vi "RT Loop - System Health and Monitoring.vi"(11 "Message Queue":refnum<queue> caption="消息队列") -> ()   [LabVIEW 2013]
uses:
  support/Message Queue/Message Cluster.ctl
  Globals/Global - Configuration Options.vi
  <vilib>/nisyscfg/Close (System).vi
  Globals/Global - All RT Loop Stop.vi
  Globals/Global - Monitoring Variables.vi
  <vilib>/NI_Real-Time Target Support.lvlib
  <vilib>/nisyscfg/nisyscfg.lvlib
  <resource>/objmgr/nisysapi.rc
  support/Message Queue/Message Queue.lvlib
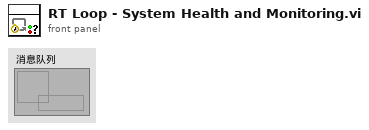
[diagram p1: front panel]
types:
  T1 = typedef "NI_Real-Time Target Support.lvlib/RT CPU Load.ctl" = cluster{"Total (%)":dbl, "Time Critical (%)":dbl, "Timed Structures (%)":dbl, "High (%)":dbl, "Above Normal (%)":dbl, "Normal (%)":dbl, "Background (%)":dbl, "Idle (%)":dbl, "ISR (%)":dbl}
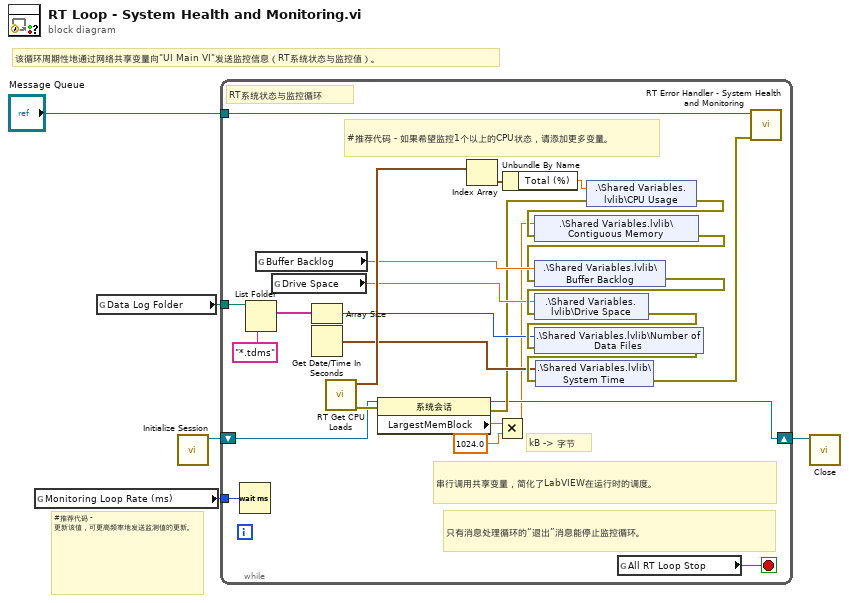
[diagram p0: block diagram]
diagram:
  # "#推荐代码 - 更新该值，可更高频率地发送监测值的更新。"
  # "该循环周期性地通过网络共享变量向\"UI Main VI\"发送监控信息（RT系统状态与监控值）。"
  n1 = global read "Global - Configuration Options.vi" "Monitoring Loop Rate (ms)"() -> (w4:u32)
  n2 = global read "Global - Configuration Options.vi" "Data Log Folder"() -> (w3:path)
  n3 = call <vilib>:"Initialize Session.vi"() -> ("session out"=w2:refnum<k21>)  [unwired: 10 in, 1 out]
  n4 = while {
    tunnel: "Message Queue" -> [w28]
    tunnel: w4 -> [w27]
    tunnel: w3 -> [w20]
    shift-right: [w10] -> w1
    shift-left: w2 -> [w9]
    stop <- w29 stop-if-true
    # "kB -> 字节"
    # "串行调用共享变量，简化了LabVIEW在运行时的调度。"
    # "#推荐代码 - 如果希望监控1个以上的CPU状态，请添加更多变量。"
    # "只有消息处理循环的“退出”消息能停止监控循环。"
    # "RT系统状态与监控循环"
    n5 = Wait (ms)(milliseconds to wait=w27) -> ()  [unwired: 1 out]
    n6 = List Folder(path=w20, pattern="*.tdms") -> (filenames=w18:string[])  [unwired: 2 in, 3 out]
    n7 = global read "Global - Monitoring Variables.vi" "Buffer Backlog"() -> (w25:dbl)
    n8 = global read "Global - Monitoring Variables.vi" "Drive Space"() -> (w22:dbl)
    n9 = Array Size(array=w18) -> (size(s)=w17:i32)
    n10 = Get Date/Time In Seconds() -> (seconds since 1Jan1904=w14:timestamp)
    n11 = call <vilib>:"RT Get CPU Loads.vi"() -> ("error out"=w12:errorcluster, "CPU loads"=w31:T1[])  [unwired: 10 in]
    n12 = property class="系统会话"(reference=w9, error in=w12) -> (reference out=w10:refnum<k21>, error out=w11:errorcluster, "LargestMemBlock"=w7:dbl)
    n13 = Index Array(array=w31) -> (element=w30:T1)  [unwired: 1 in]
    n14 = Multiply(x=w7, y=1024.0) -> (x*y=w8:dbl)
    n15 = Unbundle By Name(w30) -> ("Total (%)"=w24:dbl)
    n16 = shared-variable ".\\Shared Variables.lvlib\\CPU Usage"(w24, error in=w11) -> (error out=w26:errorcluster)
    n17 = shared-variable ".\\Shared Variables.lvlib\\Contiguous Memory"(w8, error in=w26) -> (error out=w13:errorcluster)
    n18 = shared-variable ".\\Shared Variables.lvlib\\Buffer Backlog"(w25, error in=w13) -> (error out=w23:errorcluster)
    n19 = shared-variable ".\\Shared Variables.lvlib\\Drive Space"(w22, error in=w23) -> (error out=w21:errorcluster)
    n20 = shared-variable ".\\Shared Variables.lvlib\\Number of Data Files"(w17, error in=w21) -> (error out=w16:errorcluster)
    n21 = shared-variable ".\\Shared Variables.lvlib\\System Time"(w14, error in=w16) -> (error out=w15:errorcluster)
    n22 = global read "Global - All RT Loop Stop.vi" "All RT Loop Stop"() -> (w29:bool)
    n23 = call "RT Error Handler - System Health and Monitoring.vi"("error in (no error)"=w15, "Message Queue"=w28) -> ()  [unwired: 9 in, 1 out]
  }
  n24 = call-poly <vilib>:"Close.vi"("session in"=w1) -> ()  [unwired: 10 in, 1 out]
